vi "4000_tx_rx_(chksum).vi"(0 "Write String":string="#FC", 1 "Timeout/ms":u32=300, 2 "Channel Name":string, 3 "Port Name":string, 4 "Timeout/ms Short":u32=45) -> (5 "Read":string=">+00.000", 6 "millisecond timer value":u32, 7 "Comment out":string)   [LabVIEW 2021]
panel:
  out "Raw String":string="This is simulation mode"
  in  "useChecksum":bool=TRUE
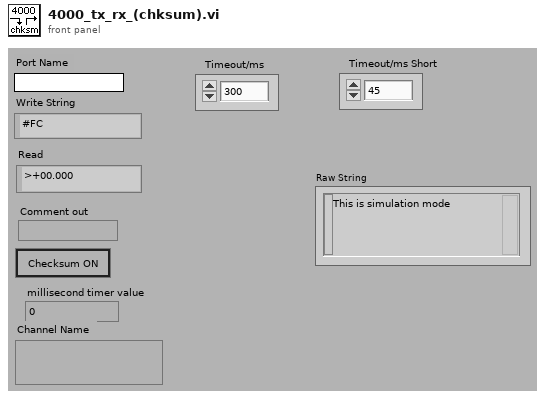
[diagram p1: front panel]
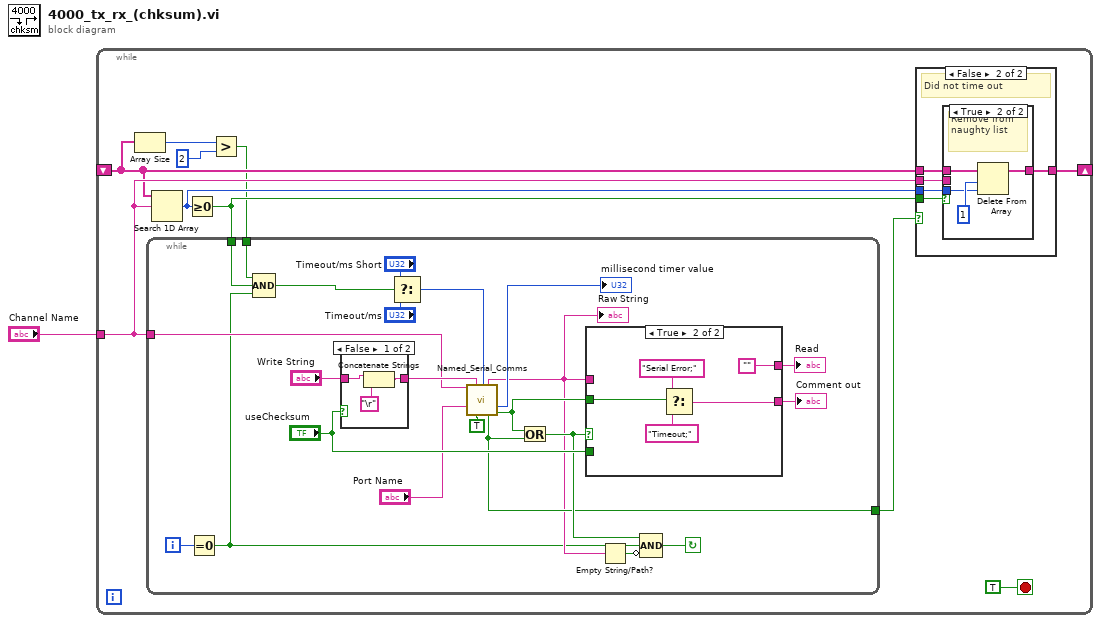
[diagram p0: block diagram]
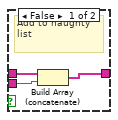
[diagram p3: hidden frame]
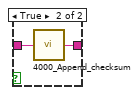
[diagram p5: hidden frame]
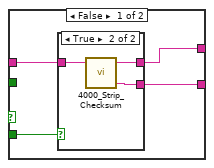
[diagram p6: hidden frame]
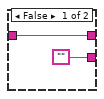
[diagram p7: hidden frame]
diagram:
  n1 = while {
    tunnel: "Channel Name" -> [w10]
    shift-right: [w9] -> _
    shift-left: _ -> [w5]
    stop <- TRUE stop-if-true
    n2 = Array Size(array=w5) -> (size(s)=w4:i32)
    n3 = Search 1D Array(1D array=w5, element=w10) -> (index of element=w6:i32)  [unwired: 1 in]
    n4 = Greater Or Equal To 0?(x=w6) -> (x >= 0?=w7:bool)
    n5 = Greater?(x=w4, y=2) -> (0:w2:bool)
    n6 = while {
      tunnel: w10 -> [w43]
      tunnel: [w42] -> w11
      tunnel: w7 -> [w37]
      tunnel: w2 -> [w30]
      i -> [w38]
      stop <- w41 continue-if-true
      n7 = Equal To 0?(x=w38) -> (x = 0?=w32:bool)
      n8 = Compound Arithmetic op=AND(w30, w37, w32) -> (w36:bool)
      n9 = case shown="False" "useChecksum" {
        tunnel: [w54 w57] -> w46
        tunnel: "Write String" -> [w55 w56]
        frame False {
          n10 = Concatenate Strings(w55, "\r") -> (w54:string)
        }
        frame True {
          n11 = call "4000_Append_checksum.vi"("ADAM command"=w56) -> ("ADAM string to send"=w57:string)
        }
      }
      n12 = Select(t="Timeout/ms Short", s=w36, f="Timeout/ms") -> (s? t:f=w35:u32)
      n13 = call "Named_Serial_Comms.vi"("Channel Name"=w43, "Write"=w46, "Timeout/ms"=w35, "Port Name"="Port Name", "Log Errors?"=TRUE) -> ("Read"=w34:string, "millisecond timer value"=→"millisecond timer value":u32, "Timed out"=w42:bool, "Serial Error"=w49:bool)  [unwired: 4 in, 3 out]
      "Raw String" <- w34
      n14 = Or(x=w49, y=w42) -> (x .or. y?=w44:bool)
      n15 = case shown="True" w44 {
        tunnel: w34 -> [w61 _]
        tunnel: [w60 w70] -> w51
        tunnel: [w59 ""] -> w50
        tunnel: w49 -> [_ w71]
        tunnel: "useChecksum" -> [w58 _]
        frame False {
          n16 = case shown="True" w58 {
            tunnel: w61 -> [w63 w66]
            tunnel: ["" w65] -> w60
            tunnel: [w63 w64] -> w59
            frame False {
            }
            frame True {
              n17 = call "4000_Strip_Checksum.vi"("ADAM response"=w66) -> ("Comment out"=w65:string, "ADAM reading"=w64:string)  [unwired: 3 out]
            }
          }
        }
        frame True {
          n18 = Select(t="Serial Error;", s=w71, f="Timeout;") -> (s? t:f=w70:string)
        }
      }
      "Read" <- w50
      "Comment out" <- w51
      n19 = Empty String/Path?(string/path=w34) -> (empty?=w33:bool)
      n20 = Compound Arithmetic op=AND(w44, w32, invert w33) -> (w41:bool)
    }
    n21 = case shown="False" w11 {
      tunnel: w7 -> [w15 w24]
      tunnel: w5 -> [w14 w23]
      tunnel: w10 -> [w13 w22]
      tunnel: [w12 w21] -> w9
      tunnel: w6 -> [_ w20]
      frame True {
        # "Channel timed out"
        n22 = case shown="True" w15 {
          tunnel: w14 -> [w18 w19]
          tunnel: w13 -> [w17 _]
          tunnel: [w16 w19] -> w12
          frame False {
            # "Add to naughty list"
            n23 = Build Array (concatenate)(w18, w17) -> (w16:string[])
          }
          frame True {
            # "Has timed out before"
          }
        }
      }
      frame False {
        # "Did not time out"
        n24 = case shown="True" w24 {
          tunnel: w23 -> [w25 w29]
          tunnel: w22 -> [_ _]
          tunnel: [w25 w27] -> w21
          tunnel: w20 -> [_ w26]
          frame False {
            # "Was not naughty"
          }
          frame True {
            # "Remove from naughty list"
            n25 = Delete From Array(array=w29, length=1, index=w26) -> (array with subset deleted=w27:string[])  [unwired: 1 out]
          }
        }
      }
    }
  }
